vi "Bar Code Reader_v4.vi"() -> ()   [LabVIEW 2016]
uses:
  <vilib>/NXT/Block Support/NXT_OutputPort.ctl
  <vilib>/NXT/Block Support/NXT_InputPort.ctl
  <vilib>/NXT/Dual Mode Library/Sensors/EV3_Color_Color.vi
  <vilib>/NXT/NXTIO Xnodes/NXTIONodeSubVIs/NXTMoveMotors.vi
  <vilib>/NXT/NXTIO Xnodes/NXTIONodeSubVIs/NXTMotorRunDistance.vi
  <vilib>/NXT/Dual Mode Library/Waits/Wait_Num.vi
  <vilib>/NXT/Subs/LVHSConnector.ctl
  <vilib>/NXT/NXTIO Xnodes/AddressXNode/NXTIOAddress.xnode
  <vilib>/NXT/NXTIO Xnodes/NXTIOXNode/NXTIO.xnode
  <vilib>/NXT/LegoClasses/BrickReference/BrickReference.lvclass
panel:
  out "Error Message":string
  out "Total Marbles":dbl
  out "Small/HDPE 4":dbl
  out "Large/Steel 4":dbl
  out "Material 4":string
  out "Small/HDPE 3":dbl
  out "Large/Steel 3":dbl
  out "Material 3":string
  out "Small/HDPE 2":dbl
  out "Large/Steel 2":dbl
  out "Material 2":string
  out "Small/HDPE 1":dbl
  out "Large/Steel 1":dbl
  out "String 3":string
  out "String 2":string
  out "Material 1":string
  out "String":string
  out "Numeric":dbl
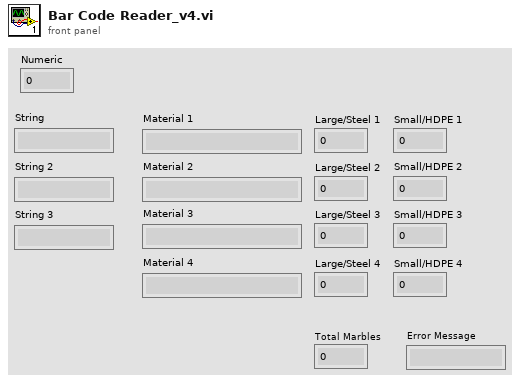
[diagram p1: front panel]
types:
  T1 = typedef "ColorSensorColors.ctl" = enum16{"No Color", "Black", "Blue", "Green", "Yellow", "Red", "White", "Brown"}
  T2 = typedef "NXT_OutputPort.ctl" = u8
  T3 = typedef "LVHSConnector.ctl" = refnum<class "BrickReference.lvclass">
  T4 = typedef "NXT_InputPort.ctl" = u32
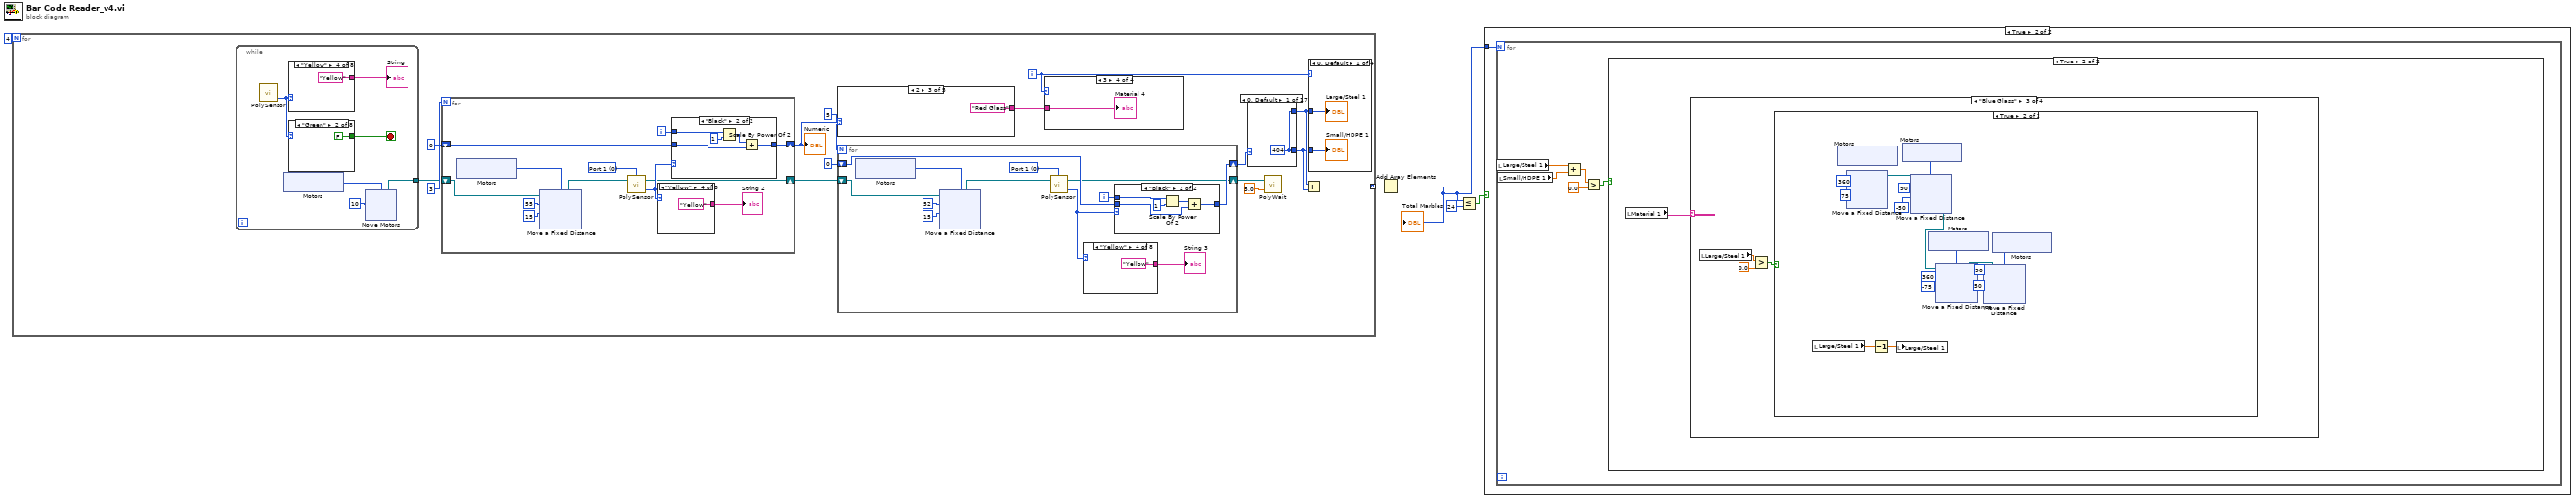
[diagram p0: block diagram]
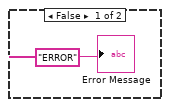
[diagram p2: hidden frame]
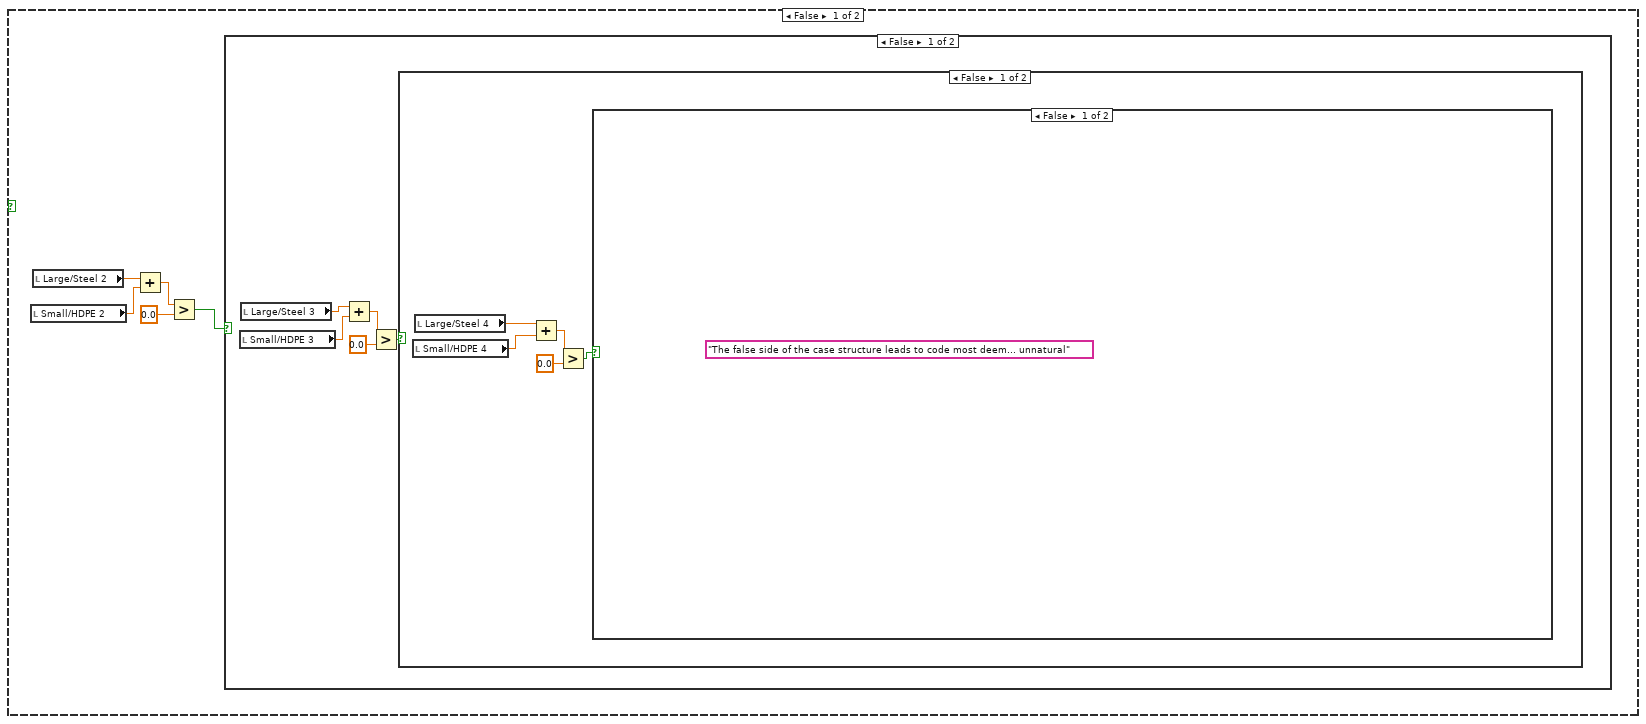
[diagram p3: hidden frame]
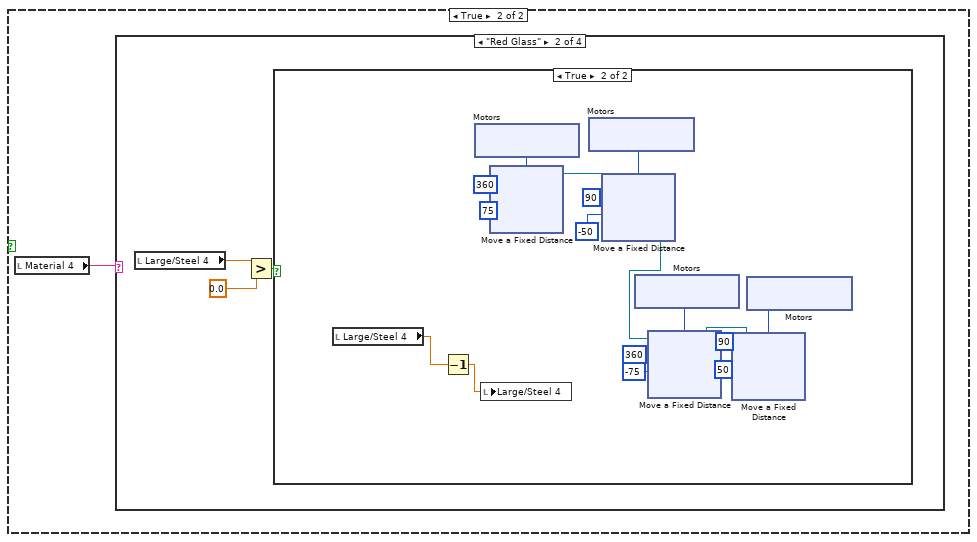
[diagram p4: hidden frame]
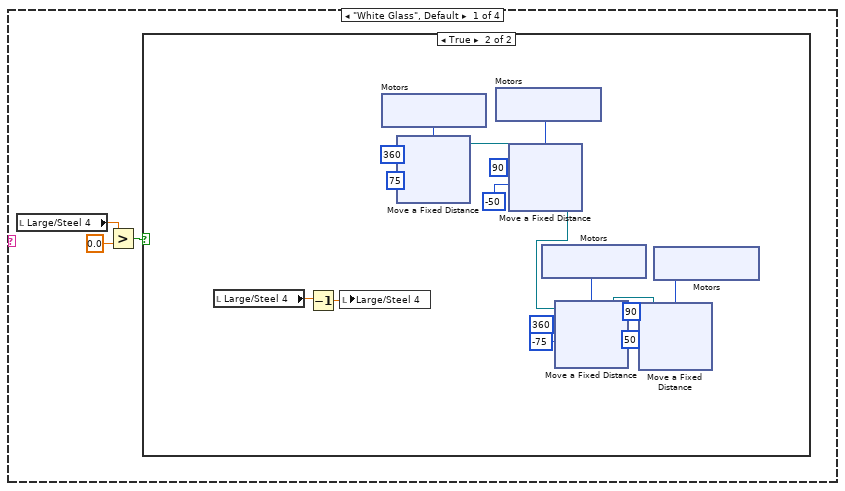
[diagram p5: hidden frame]
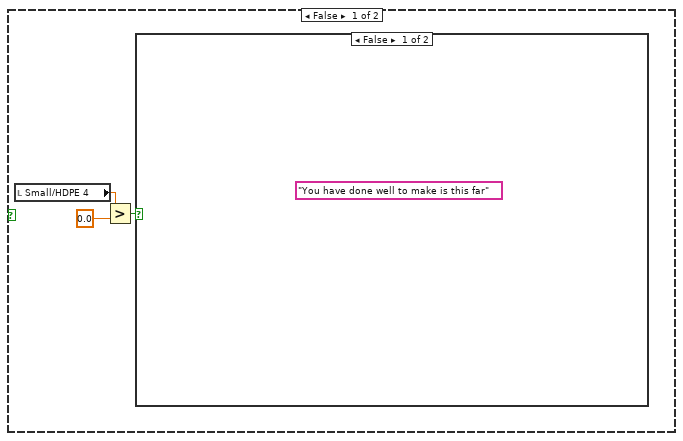
[diagram p6: hidden frame]
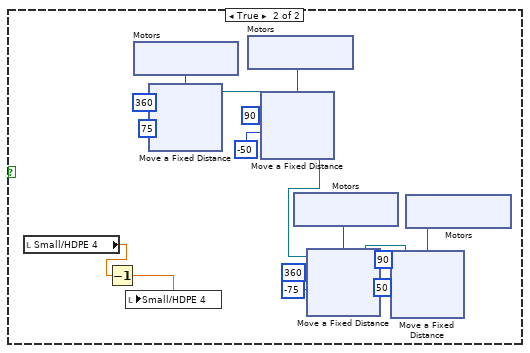
[diagram p7: hidden frame]
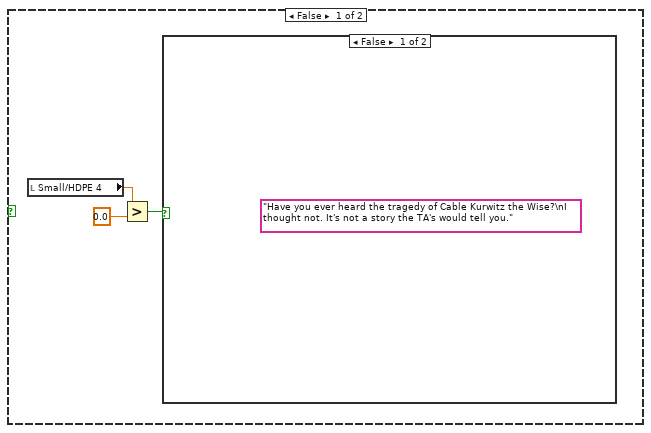
[diagram p8: hidden frame]
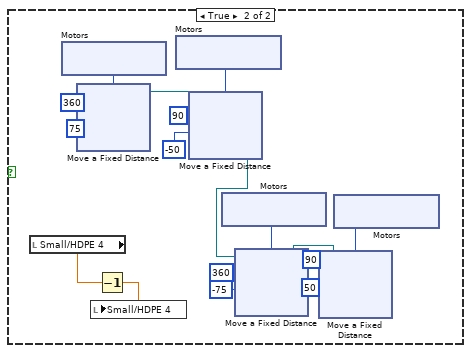
[diagram p9: hidden frame]
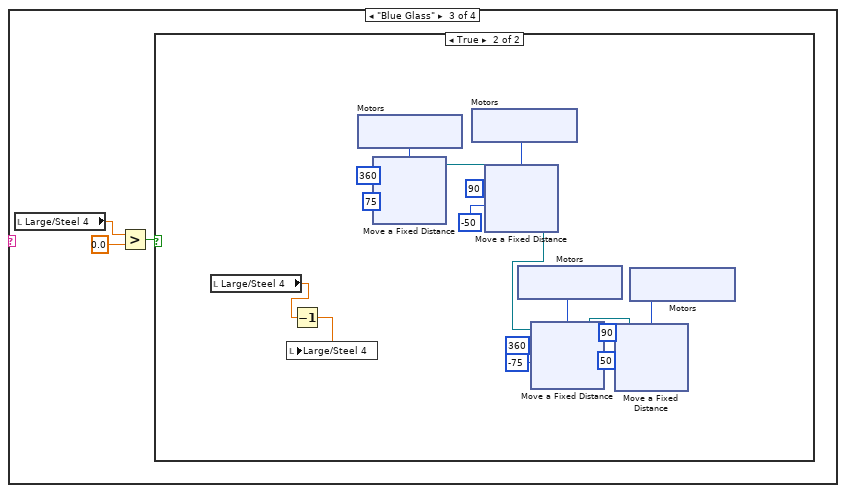
[diagram p10: hidden frame]
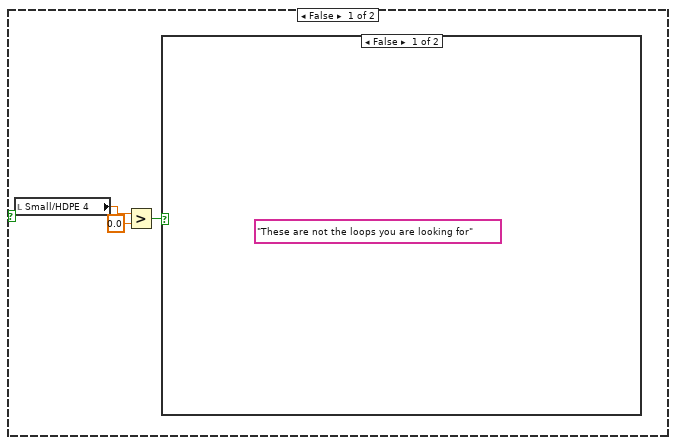
[diagram p11: hidden frame]
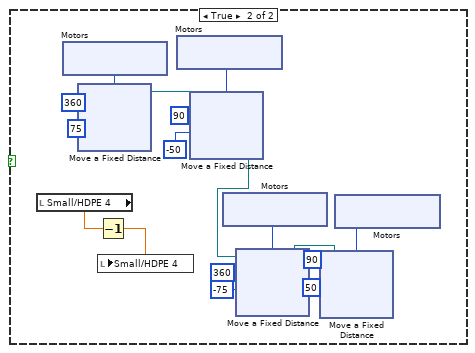
[diagram p12: hidden frame]
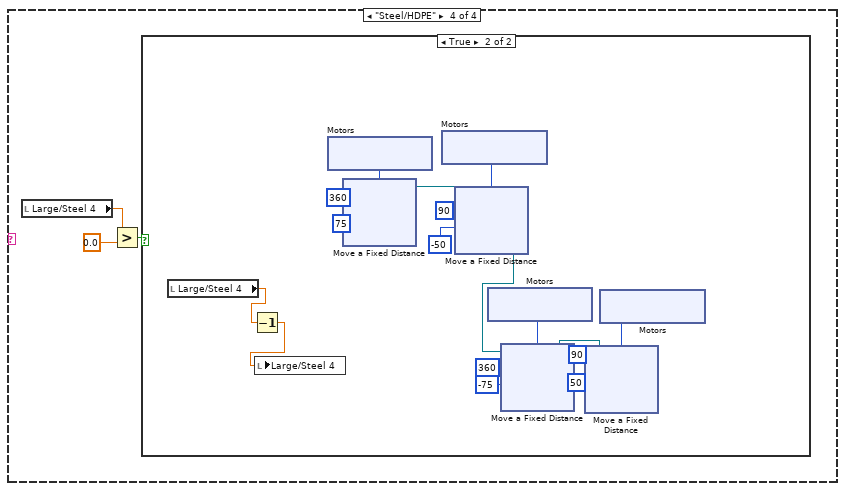
[diagram p13: hidden frame]
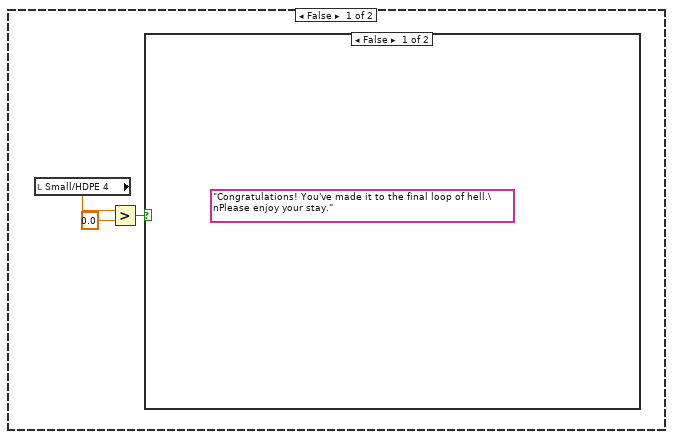
[diagram p14: hidden frame]
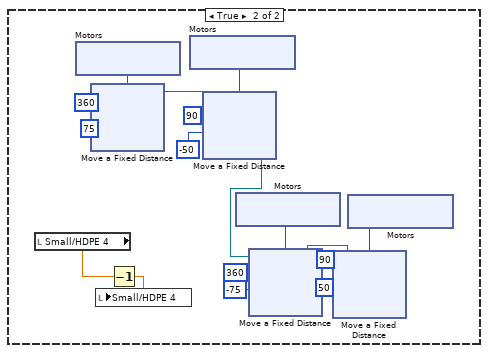
[diagram p15: hidden frame]
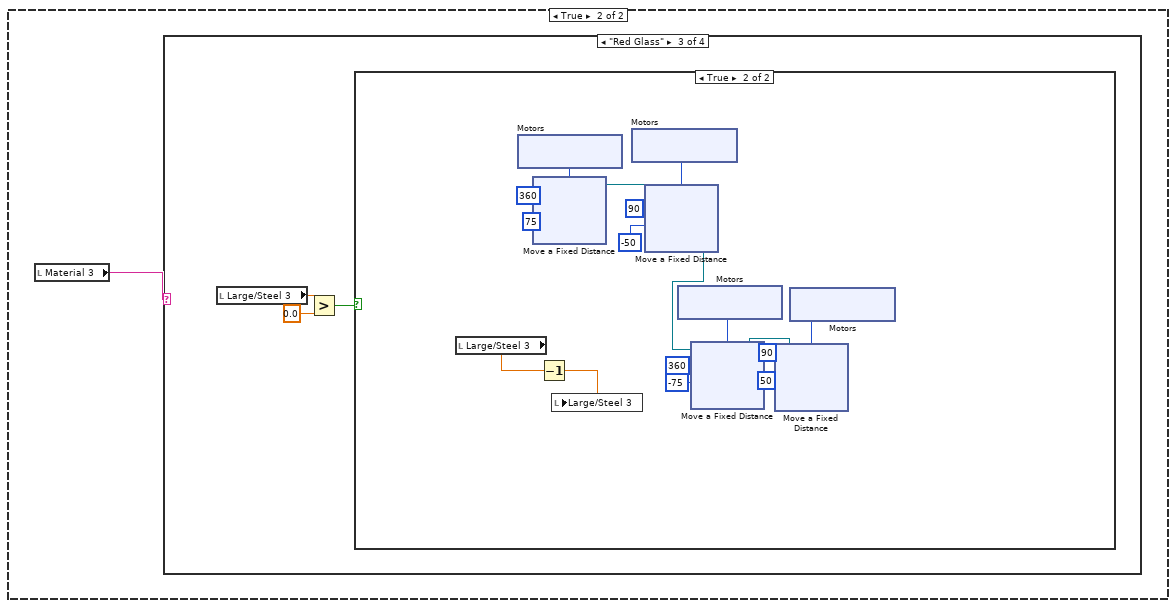
[diagram p16: hidden frame]
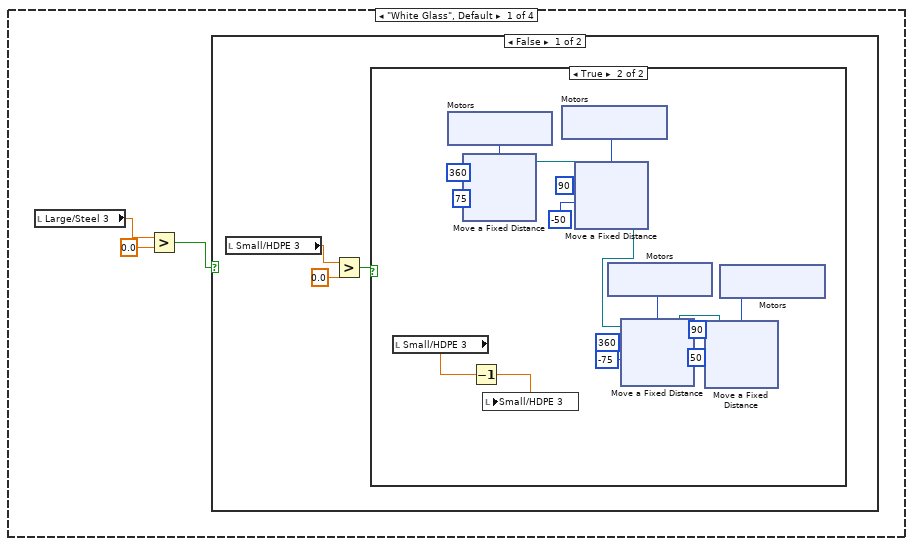
[diagram p17: hidden frame]
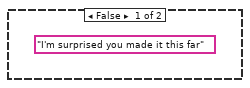
[diagram p18: hidden frame]
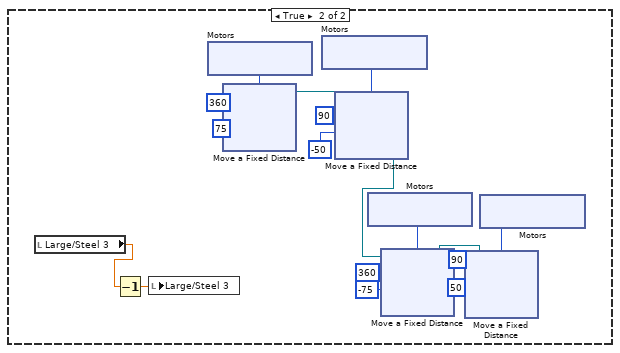
[diagram p19: hidden frame]
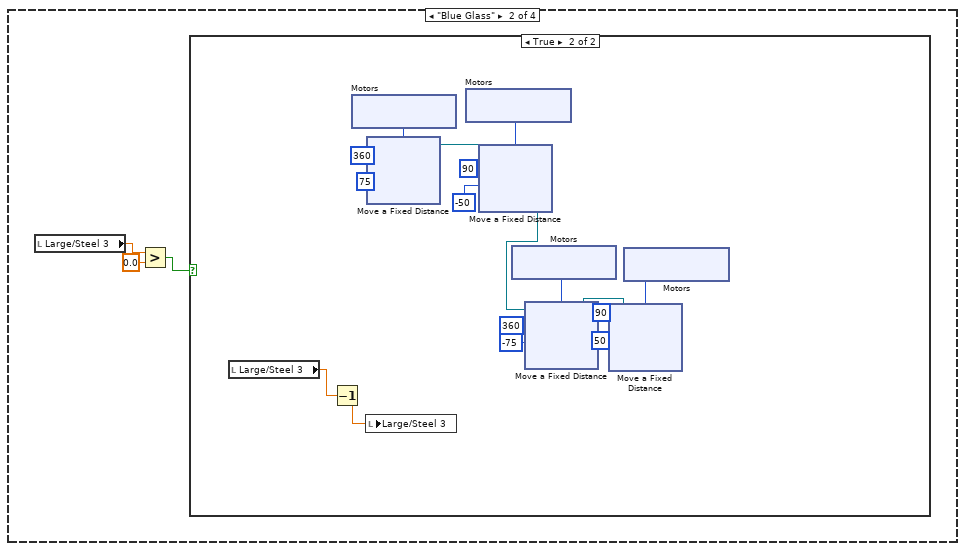
[diagram p20: hidden frame]
diagram:
  n1 = for {
    N: 4 -> [_]
    tunnel: [w6] -> w4 mode=indexing
    i -> [w11]
    n2 = while {
      tunnel: [w109] -> w18
      stop <- w113 stop-if-true
      n3 = call-poly <vilib>:"PolySensor.vi"() -> ("Detected Color"=w111:T1)  [unwired: 3 in, 1 out]
      n4 = xnode "Motors"() -> ("Motor"=w108:T2)
      n5 = case shown="\"Yellow\"" w111 {
        tunnel: ["No Color" "Blue" "Green" "Yellow" "Red" "White" "Brown" "Black"] -> w112
        frame "No Color", Default {
        }
        frame "Blue" {
        }
        frame "Green" {
        }
        frame "Yellow" {
        }
        frame "Red" {
        }
        frame "White" {
        }
        frame "Brown" {
        }
        frame "Black" {
        }
      }
      "String" <- w112
      n6 = case shown="\"Green\"" w111 {
        tunnel: [FALSE FALSE FALSE FALSE FALSE FALSE FALSE TRUE] -> w113
        frame "No Color", Default {
        }
        frame "Green" {
        }
        frame "Yellow" {
        }
        frame "Red" {
        }
        frame "White" {
        }
        frame "Brown" {
        }
        frame "Blue" {
        }
        frame "Black" {
        }
      }
      n7 = xnode "Move Motors"("Power/Speed 1"=i8 10, "Motors"=w108) -> ("NXT/EV3"=w109:T3)  [unwired: 1 in]
    }
    n8 = for {
      N: 3 -> [_]
      shift-right: [w149] -> w17
      shift-left: 0 -> [w148]
      shift-right: [w144] -> w13
      shift-left: w18 -> [w141]
      i -> [w145]
      w138 = T4 0 items=["Port 1", "Port 2", "Port 3", "Port 4"] ("Port (Port 1)")
      n9 = xnode "Motors"() -> ("Motor"=w139:T2)
      n10 = xnode "Move a Fixed Distance"("Speed 1"=i8 15, "Distance 1"=55, "Motors"=w139, "NXT/EV3"=w141) -> ("NXT/EV3"=w140:T3)
      n11 = call-poly <vilib>:"PolySensor.vi"("NXT/EV3"=w140, "Port (Port 1)"=w138) -> ("Detected Color"=w146:T1, "NXT/EV3"=w144:T3)  [unwired: 1 in]
      n12 = case shown="\"Yellow\"" w146 {
        tunnel: ["No Color" "Blue" "Green" "Yellow" "Red" "White" "Brown" "Black"] -> w147
        frame "No Color", Default {
        }
        frame "Blue" {
        }
        frame "Green" {
        }
        frame "Yellow" {
        }
        frame "Red" {
        }
        frame "White" {
        }
        frame "Brown" {
        }
        frame "Black" {
        }
      }
      "String 2" <- w147
      n13 = case shown="\"Black\"" w146 {
        tunnel: w145 -> [_ w173]
        tunnel: [w169 w171] -> w149
        tunnel: w148 -> [w169 w170]
        frame "White", Default {
        }
        frame "Black" {
          n14 = Scale By Power Of 2(n=w173, x=1) -> (x*2^n=w172:i32)
          n15 = Add(x=w172, y=w170) -> (x+y=w171:i32)
        }
      }
    }
    "Numeric" <- w17
    n16 = case shown="2" w17 {
      tunnel: ["Something has gone wrong" "White Glass" "Red Glass" "Blue Glass" "Steel/HDPE"] -> w16
      frame 0, Default {
      }
      frame 1 {
      }
      frame 2 {
      }
      frame 3 {
      }
      frame 4 {
      }
    }
    n17 = for {
      N: 5 -> [_]
      shift-right: [w77] -> w12
      shift-left: 0 -> [w76]
      shift-right: [w72] -> w10
      shift-left: w13 -> [w69]
      i -> [w73]
      w66 = T4 0 items=["Port 1", "Port 2", "Port 3", "Port 4"] ("Port (Port 1)")
      n18 = xnode "Motors"() -> ("Motor"=w67:T2)
      n19 = xnode "Move a Fixed Distance"("Speed 1"=i8 15, "Distance 1"=52, "Motors"=w67, "NXT/EV3"=w69) -> ("NXT/EV3"=w68:T3)
      n20 = call-poly <vilib>:"PolySensor.vi"("NXT/EV3"=w68, "Port (Port 1)"=w66) -> ("Detected Color"=w74:T1, "NXT/EV3"=w72:T3)  [unwired: 1 in]
      n21 = case shown="\"Yellow\"" w74 {
        tunnel: ["No Color" "Blue" "Green" "Yellow" "Red" "White" "Brown" "Black"] -> w75
        frame "No Color", Default {
        }
        frame "Blue" {
        }
        frame "Green" {
        }
        frame "Yellow" {
        }
        frame "Red" {
        }
        frame "White" {
        }
        frame "Brown" {
        }
        frame "Black" {
        }
      }
      "String 3" <- w75
      n22 = case shown="\"Black\"" w74 {
        tunnel: w73 -> [_ w101]
        tunnel: [w97 w99] -> w77
        tunnel: w76 -> [w97 w98]
        frame "White", Default {
        }
        frame "Black" {
          n23 = Scale By Power Of 2(n=w101, x=1) -> (x*2^n=w100:i32)
          n24 = Add(x=w100, y=w98) -> (x+y=w99:i32)
        }
      }
    }
    n25 = case shown="3" w11 {
      tunnel: w16 -> [w29 w30 w31 w32]
      frame 0, Default {
        "Material 1" <- w29
      }
      frame 1 {
        "Material 2" <- w30
      }
      frame 2 {
        "Material 3" <- w31
      }
      frame 3 {
        "Material 4" <- w32
      }
    }
    n26 = case shown="0, Default" w12 {
      tunnel: [w33 0 1 2 3 0 1 2 3 0 1 2 3 0 1 2 3] -> w8
      tunnel: [w33 0 0 0 0 1 1 1 1 2 2 2 2 3 3 3 3] -> w7
      frame 0, Default {
        w33 = 404
      }
      frame 1 {
      }
      frame 2 {
      }
      frame 3 {
      }
      frame 4 {
      }
      frame 5 {
      }
      frame 6 {
      }
      frame 7 {
      }
      frame 8 {
      }
      frame 9 {
      }
      frame 10 {
      }
      frame 11 {
      }
      frame 12 {
      }
      frame 13 {
      }
      frame 14 {
      }
      frame 15 {
      }
      frame 16 {
      }
    }
    n27 = call-poly <vilib>:"PolyWait.vi"("Time (1 sec)"=sgl 5.0, "NXT/EV3"=w10) -> ()  [unwired: 2 in, 1 out]
    n28 = Add(x=w8, y=w7) -> (x+y=w6:i32)
    n29 = case shown="0, Default" w11 {
      tunnel: w8 -> [w22 w23 w25 w27]
      tunnel: w7 -> [w21 w24 w26 w28]
      frame 0, Default {
        "Small/HDPE 1" <- w21
        "Large/Steel 1" <- w22
      }
      frame 1 {
        "Large/Steel 2" <- w23
        "Small/HDPE 2" <- w24
      }
      frame 2 {
        "Large/Steel 3" <- w25
        "Small/HDPE 3" <- w26
      }
      frame 3 {
        "Large/Steel 4" <- w27
        "Small/HDPE 4" <- w28
      }
    }
  }
  n30 = Add Array Elements(numeric array=w4) -> (sum=w3:i32)
  "Total Marbles" <- w3
  n31 = Less Or Equal?(x=w3, y=24) -> (x <= y?=w1:bool)
  n32 = case shown="True" w1 {
    tunnel: w3 -> [_ w176]
    frame False {
      "Error Message" <- "ERROR"
    }
    frame True {
      n33 = for {
        N: w176 -> [_]
        n34 = local read "Large/Steel 1"() -> (w181:dbl)
        n35 = local read "Small/HDPE 1"() -> (w180:dbl)
        n36 = Add(x=w181, y=w180) -> (x+y=w179:dbl)
        n37 = Greater?(x=w179, y=0.0) -> (0:w177:bool)
        n38 = case shown="True" w177 {
          frame False {
            n39 = local read "Small/HDPE 2"() -> (w184:dbl)
            n40 = local read "Large/Steel 2"() -> (w183:dbl)
            n41 = Add(x=w183, y=w184) -> (x+y=w186:dbl)
            n42 = Greater?(x=w186, y=0.0) -> (0:w182:bool)
            n43 = case shown="False" w182 {
              frame False {
                n44 = local read "Small/HDPE 3"() -> (w188:dbl)
                n45 = local read "Large/Steel 3"() -> (w189:dbl)
                n46 = Add(x=w189, y=w188) -> (x+y=w191:dbl)
                n47 = Greater?(x=w191, y=0.0) -> (0:w187:bool)
                n48 = case shown="False" w187 {
                  frame False {
                    n49 = local read "Small/HDPE 4"() -> (w193:dbl)
                    n50 = local read "Large/Steel 4"() -> (w194:dbl)
                    n51 = Add(x=w194, y=w193) -> (x+y=w196:dbl)
                    n52 = Greater?(x=w196, y=0.0) -> (0:w192:bool)
                    n53 = case shown="False" w192 {
                      frame False {
                        (unwired) "The false side of the case structure leads to code most deem... unnatural"
                      }
                      frame True {
                        n54 = local read "Material 4"() -> (w197:string)
                        n55 = case shown="\"Red Glass\"" w197 {
                          frame "White Glass", Default {
                            n56 = local read "Large/Steel 4"() -> (w199:dbl)
                            n57 = Greater?(x=w199, y=0.0) -> (0:w200:bool)
                            n58 = case shown="True" w200 {
                              frame False {
                                n59 = local read "Small/HDPE 4"() -> (w202:dbl)
                                n60 = Greater?(x=w202, y=0.0) -> (0:w203:bool)
                                n61 = case shown="False" w203 {
                                frame False {
                                (unwired) "You have done well to make is this far"
                                }
                                frame True {
                                n62 = local read "Small/HDPE 4"() -> (w220:dbl)
                                n63 = Decrement(x=w220) -> (x-1=w219:dbl)
                                n64 = local write "Small/HDPE 4"(w219) -> ()
                                n65 = xnode "Motors"() -> ("Motor"=w204:T2)
                                n66 = xnode "Move a Fixed Distance"("Speed 1"=i8 75, "Distance 1"=360, "Motors"=w204) -> ("NXT/EV3"=w207:T3)  [unwired: 1 in]
                                n67 = xnode "Motors"() -> ("Motor"=w208:T2)
                                n68 = xnode "Move a Fixed Distance"("Speed 1"=i8 -50, "Distance 1"=90, "Motors"=w208, "NXT/EV3"=w207) -> ("NXT/EV3"=w218:T3)
                                n69 = xnode "Motors"() -> ("Motor"=w214:T2)
                                n70 = xnode "Move a Fixed Distance"("Speed 1"=i8 -75, "Distance 1"=360, "Motors"=w214, "NXT/EV3"=w218) -> ("NXT/EV3"=w217:T3)
                                n71 = xnode "Motors"() -> ("Motor"=w211:T2)
                                n72 = xnode "Move a Fixed Distance"("Speed 1"=i8 50, "Distance 1"=90, "Motors"=w211, "NXT/EV3"=w217) -> ()  [unwired: 1 out]
                                }
                                }
                              }
                              frame True {
                                n73 = local read "Large/Steel 4"() -> (w281:dbl)
                                n74 = Decrement(x=w281) -> (x-1=w280:dbl)
                                n75 = local write "Large/Steel 4"(w280) -> ()
                                n76 = xnode "Motors"() -> ("Motor"=w265:T2)
                                n77 = xnode "Move a Fixed Distance"("Speed 1"=i8 75, "Distance 1"=360, "Motors"=w265) -> ("NXT/EV3"=w268:T3)  [unwired: 1 in]
                                n78 = xnode "Motors"() -> ("Motor"=w269:T2)
                                n79 = xnode "Move a Fixed Distance"("Speed 1"=i8 -50, "Distance 1"=90, "Motors"=w269, "NXT/EV3"=w268) -> ("NXT/EV3"=w279:T3)
                                n80 = xnode "Motors"() -> ("Motor"=w275:T2)
                                n81 = xnode "Move a Fixed Distance"("Speed 1"=i8 -75, "Distance 1"=360, "Motors"=w275, "NXT/EV3"=w279) -> ("NXT/EV3"=w278:T3)
                                n82 = xnode "Motors"() -> ("Motor"=w272:T2)
                                n83 = xnode "Move a Fixed Distance"("Speed 1"=i8 50, "Distance 1"=90, "Motors"=w272, "NXT/EV3"=w278) -> ()  [unwired: 1 out]
                              }
                            }
                          }
                          frame "Red Glass" {
                            n84 = local read "Large/Steel 4"() -> (w327:dbl)
                            n85 = Greater?(x=w327, y=0.0) -> (0:w328:bool)
                            n86 = case shown="True" w328 {
                              frame False {
                                n87 = local read "Small/HDPE 4"() -> (w329:dbl)
                                n88 = Greater?(x=w329, y=0.0) -> (0:w331:bool)
                                n89 = case shown="False" w331 {
                                frame False {
                                (unwired) "Have you ever heard the tragedy of Cable Kurwitz the Wise?\nI thought not. It's not a story the TA's would tell you."
                                }
                                frame True {
                                n90 = local read "Small/HDPE 4"() -> (w348:dbl)
                                n91 = xnode "Motors"() -> ("Motor"=w332:T2)
                                n92 = xnode "Move a Fixed Distance"("Speed 1"=i8 75, "Distance 1"=360, "Motors"=w332) -> ("NXT/EV3"=w335:T3)  [unwired: 1 in]
                                n93 = Decrement(x=w348) -> (x-1=w347:dbl)
                                n94 = local write "Small/HDPE 4"(w347) -> ()
                                n95 = xnode "Motors"() -> ("Motor"=w336:T2)
                                n96 = xnode "Move a Fixed Distance"("Speed 1"=i8 -50, "Distance 1"=90, "Motors"=w336, "NXT/EV3"=w335) -> ("NXT/EV3"=w346:T3)
                                n97 = xnode "Motors"() -> ("Motor"=w342:T2)
                                n98 = xnode "Move a Fixed Distance"("Speed 1"=i8 -75, "Distance 1"=360, "Motors"=w342, "NXT/EV3"=w346) -> ("NXT/EV3"=w345:T3)
                                n99 = xnode "Motors"() -> ("Motor"=w339:T2)
                                n100 = xnode "Move a Fixed Distance"("Speed 1"=i8 50, "Distance 1"=90, "Motors"=w339, "NXT/EV3"=w345) -> ()  [unwired: 1 out]
                                }
                                }
                              }
                              frame True {
                                n101 = local read "Large/Steel 4"() -> (w409:dbl)
                                n102 = Decrement(x=w409) -> (x-1=w408:dbl)
                                n103 = xnode "Motors"() -> ("Motor"=w393:T2)
                                n104 = local write "Large/Steel 4"(w408) -> ()
                                n105 = xnode "Move a Fixed Distance"("Speed 1"=i8 75, "Distance 1"=360, "Motors"=w393) -> ("NXT/EV3"=w396:T3)  [unwired: 1 in]
                                n106 = xnode "Motors"() -> ("Motor"=w397:T2)
                                n107 = xnode "Move a Fixed Distance"("Speed 1"=i8 -50, "Distance 1"=90, "Motors"=w397, "NXT/EV3"=w396) -> ("NXT/EV3"=w407:T3)
                                n108 = xnode "Motors"() -> ("Motor"=w403:T2)
                                n109 = xnode "Move a Fixed Distance"("Speed 1"=i8 -75, "Distance 1"=360, "Motors"=w403, "NXT/EV3"=w407) -> ("NXT/EV3"=w406:T3)
                                n110 = xnode "Motors"() -> ("Motor"=w400:T2)
                                n111 = xnode "Move a Fixed Distance"("Speed 1"=i8 50, "Distance 1"=90, "Motors"=w400, "NXT/EV3"=w406) -> ()  [unwired: 1 out]
                              }
                            }
                          }
                          frame "Blue Glass" {
                            n112 = local read "Large/Steel 4"() -> (w456:dbl)
                            n113 = Greater?(x=w456, y=0.0) -> (0:w455:bool)
                            n114 = case shown="True" w455 {
                              frame False {
                                n115 = local read "Small/HDPE 4"() -> (w458:dbl)
                                n116 = Greater?(x=w458, y=0.0) -> (0:w459:bool)
                                n117 = case shown="False" w459 {
                                frame False {
                                (unwired) "These are not the loops you are looking for"
                                }
                                frame True {
                                n118 = local read "Small/HDPE 4"() -> (w476:dbl)
                                n119 = xnode "Motors"() -> ("Motor"=w460:T2)
                                n120 = xnode "Move a Fixed Distance"("Speed 1"=i8 75, "Distance 1"=360, "Motors"=w460) -> ("NXT/EV3"=w463:T3)  [unwired: 1 in]
                                n121 = Decrement(x=w476) -> (x-1=w475:dbl)
                                n122 = local write "Small/HDPE 4"(w475) -> ()
                                n123 = xnode "Motors"() -> ("Motor"=w464:T2)
                                n124 = xnode "Move a Fixed Distance"("Speed 1"=i8 -50, "Distance 1"=90, "Motors"=w464, "NXT/EV3"=w463) -> ("NXT/EV3"=w474:T3)
                                n125 = xnode "Motors"() -> ("Motor"=w470:T2)
                                n126 = xnode "Move a Fixed Distance"("Speed 1"=i8 -75, "Distance 1"=360, "Motors"=w470, "NXT/EV3"=w474) -> ("NXT/EV3"=w473:T3)
                                n127 = xnode "Motors"() -> ("Motor"=w467:T2)
                                n128 = xnode "Move a Fixed Distance"("Speed 1"=i8 50, "Distance 1"=90, "Motors"=w467, "NXT/EV3"=w473) -> ()  [unwired: 1 out]
                                }
                                }
                              }
                              frame True {
                                n129 = local read "Large/Steel 4"() -> (w537:dbl)
                                n130 = Decrement(x=w537) -> (x-1=w536:dbl)
                                n131 = local write "Large/Steel 4"(w536) -> ()
                                n132 = xnode "Motors"() -> ("Motor"=w521:T2)
                                n133 = xnode "Move a Fixed Distance"("Speed 1"=i8 75, "Distance 1"=360, "Motors"=w521) -> ("NXT/EV3"=w524:T3)  [unwired: 1 in]
                                n134 = xnode "Motors"() -> ("Motor"=w525:T2)
                                n135 = xnode "Move a Fixed Distance"("Speed 1"=i8 -50, "Distance 1"=90, "Motors"=w525, "NXT/EV3"=w524) -> ("NXT/EV3"=w535:T3)
                                n136 = xnode "Motors"() -> ("Motor"=w531:T2)
                                n137 = xnode "Move a Fixed Distance"("Speed 1"=i8 -75, "Distance 1"=360, "Motors"=w531, "NXT/EV3"=w535) -> ("NXT/EV3"=w534:T3)
                                n138 = xnode "Motors"() -> ("Motor"=w528:T2)
                                n139 = xnode "Move a Fixed Distance"("Speed 1"=i8 50, "Distance 1"=90, "Motors"=w528, "NXT/EV3"=w534) -> ()  [unwired: 1 out]
                              }
                            }
                          }
                          frame "Steel/HDPE" {
                            n140 = local read "Large/Steel 4"() -> (w583:dbl)
                            n141 = Greater?(x=w583, y=0.0) -> (0:w584:bool)
                            n142 = case shown="True" w584 {
                              frame False {
                                n143 = local read "Small/HDPE 4"() -> (w586:dbl)
                                n144 = Greater?(x=w586, y=0.0) -> (0:w587:bool)
                                n145 = case shown="False" w587 {
                                frame False {
                                (unwired) "Congratulations! You've made it to the final loop of hell.\nPlease enjoy your stay."
                                }
                                frame True {
                                n146 = local read "Small/HDPE 4"() -> (w604:dbl)
                                n147 = xnode "Motors"() -> ("Motor"=w588:T2)
                                n148 = xnode "Move a Fixed Distance"("Speed 1"=i8 75, "Distance 1"=360, "Motors"=w588) -> ("NXT/EV3"=w591:T3)  [unwired: 1 in]
                                n149 = Decrement(x=w604) -> (x-1=w603:dbl)
                                n150 = local write "Small/HDPE 4"(w603) -> ()
                                n151 = xnode "Motors"() -> ("Motor"=w592:T2)
                                n152 = xnode "Move a Fixed Distance"("Speed 1"=i8 -50, "Distance 1"=90, "Motors"=w592, "NXT/EV3"=w591) -> ("NXT/EV3"=w602:T3)
                                n153 = xnode "Motors"() -> ("Motor"=w598:T2)
                                n154 = xnode "Move a Fixed Distance"("Speed 1"=i8 -75, "Distance 1"=360, "Motors"=w598, "NXT/EV3"=w602) -> ("NXT/EV3"=w601:T3)
                                n155 = xnode "Motors"() -> ("Motor"=w595:T2)
                                n156 = xnode "Move a Fixed Distance"("Speed 1"=i8 50, "Distance 1"=90, "Motors"=w595, "NXT/EV3"=w601) -> ()  [unwired: 1 out]
                                }
                                }
                              }
                              frame True {
                                n157 = local read "Large/Steel 4"() -> (w665:dbl)
                                n158 = Decrement(x=w665) -> (x-1=w664:dbl)
                                n159 = local write "Large/Steel 4"(w664) -> ()
                                n160 = xnode "Motors"() -> ("Motor"=w649:T2)
                                n161 = xnode "Move a Fixed Distance"("Speed 1"=i8 75, "Distance 1"=360, "Motors"=w649) -> ("NXT/EV3"=w652:T3)  [unwired: 1 in]
                                n162 = xnode "Motors"() -> ("Motor"=w653:T2)
                                n163 = xnode "Move a Fixed Distance"("Speed 1"=i8 -50, "Distance 1"=90, "Motors"=w653, "NXT/EV3"=w652) -> ("NXT/EV3"=w663:T3)
                                n164 = xnode "Motors"() -> ("Motor"=w659:T2)
                                n165 = xnode "Move a Fixed Distance"("Speed 1"=i8 -75, "Distance 1"=360, "Motors"=w659, "NXT/EV3"=w663) -> ("NXT/EV3"=w662:T3)
                                n166 = xnode "Motors"() -> ("Motor"=w656:T2)
                                n167 = xnode "Move a Fixed Distance"("Speed 1"=i8 50, "Distance 1"=90, "Motors"=w656, "NXT/EV3"=w662) -> ()  [unwired: 1 out]
                              }
                            }
                          }
                        }
                      }
                    }
                  }
                  frame True {
                    n168 = local read "Material 3"() -> (w710:string)
                    n169 = case shown="\"Red Glass\"" w710 {
                      frame "White Glass", Default {
                        n170 = local read "Large/Steel 3"() -> (w713:dbl)
                        n171 = Greater?(x=w713, y=0.0) -> (0:w711:bool)
                        n172 = case shown="False" w711 {
                          frame False {
                            n173 = local read "Small/HDPE 3"() -> (w715:dbl)
                            n174 = Greater?(x=w715, y=0.0) -> (0:w716:bool)
                            n175 = case shown="True" w716 {
                              frame False {
                                (unwired) "I'm surprised you made it this far"
                              }
                              frame True {
                                n176 = local read "Small/HDPE 3"() -> (w733:dbl)
                                n177 = xnode "Motors"() -> ("Motor"=w717:T2)
                                n178 = xnode "Move a Fixed Distance"("Speed 1"=i8 75, "Distance 1"=360, "Motors"=w717) -> ("NXT/EV3"=w720:T3)  [unwired: 1 in]
                                n179 = Decrement(x=w733) -> (x-1=w732:dbl)
                                n180 = local write "Small/HDPE 3"(w732) -> ()
                                n181 = xnode "Motors"() -> ("Motor"=w721:T2)
                                n182 = xnode "Move a Fixed Distance"("Speed 1"=i8 -50, "Distance 1"=90, "Motors"=w721, "NXT/EV3"=w720) -> ("NXT/EV3"=w731:T3)
                                n183 = xnode "Motors"() -> ("Motor"=w727:T2)
                                n184 = xnode "Move a Fixed Distance"("Speed 1"=i8 -75, "Distance 1"=360, "Motors"=w727, "NXT/EV3"=w731) -> ("NXT/EV3"=w730:T3)
                                n185 = xnode "Motors"() -> ("Motor"=w724:T2)
                                n186 = xnode "Move a Fixed Distance"("Speed 1"=i8 50, "Distance 1"=90, "Motors"=w724, "NXT/EV3"=w730) -> ()  [unwired: 1 out]
                              }
                            }
                          }
                          frame True {
                            n187 = local read "Large/Steel 3"() -> (w794:dbl)
                            n188 = Decrement(x=w794) -> (x-1=w793:dbl)
                            n189 = local write "Large/Steel 3"(w793) -> ()
                            n190 = xnode "Motors"() -> ("Motor"=w778:T2)
                            n191 = xnode "Move a Fixed Distance"("Speed 1"=i8 75, "Distance 1"=360, "Motors"=w778) -> ("NXT/EV3"=w781:T3)  [unwired: 1 in]
                            n192 = xnode "Motors"() -> ("Motor"=w782:T2)
                            n193 = xnode "Move a Fixed Distance"("Speed 1"=i8 -50, "Distance 1"=90, "Motors"=w782, "NXT/EV3"=w781) -> ("NXT/EV3"=w792:T3)
                            n194 = xnode "Motors"() -> ("Motor"=w788:T2)
                            n195 = xnode "Move a Fixed Distance"("Speed 1"=i8 -75, "Distance 1"=360, "Motors"=w788, "NXT/EV3"=w792) -> ("NXT/EV3"=w791:T3)
                            n196 = xnode "Motors"() -> ("Motor"=w785:T2)
                            n197 = xnode "Move a Fixed Distance"("Speed 1"=i8 50, "Distance 1"=90, "Motors"=w785, "NXT/EV3"=w791) -> ()  [unwired: 1 out]
                          }
                        }
                      }
                      frame "Blue Glass" {
                        n198 = local read "Large/Steel 3"() -> (w841:dbl)
                        n199 = Greater?(x=w841, y=0.0) -> (0:w839:bool)
                        n200 = case shown="True" w839 {
                          frame False {
                            n201 = local read "Small/HDPE 3"() -> (w844:dbl)
                            n202 = Greater?(x=w844, y=0.0) -> (0:w842:bool)
                            n203 = case shown="False" w842 {
                              frame False {
                                (unwired) "Welcome to the dark side of the case structure"
                              }
                              frame True {
                                n204 = local read "Small/HDPE 3"() -> (w861:dbl)
                                n205 = xnode "Motors"() -> ("Motor"=w845:T2)
                                n206 = Decrement(x=w861) -> (x-1=w860:dbl)
                                n207 = xnode "Move a Fixed Distance"("Speed 1"=i8 75, "Distance 1"=360, "Motors"=w845) -> ("NXT/EV3"=w848:T3)  [unwired: 1 in]
                                n208 = local write "Small/HDPE 3"(w860) -> ()
                                n209 = xnode "Motors"() -> ("Motor"=w849:T2)
                                n210 = xnode "Move a Fixed Distance"("Speed 1"=i8 -50, "Distance 1"=90, "Motors"=w849, "NXT/EV3"=w848) -> ("NXT/EV3"=w859:T3)
                                n211 = xnode "Motors"() -> ("Motor"=w855:T2)
                                n212 = xnode "Move a Fixed Distance"("Speed 1"=i8 -75, "Distance 1"=360, "Motors"=w855, "NXT/EV3"=w859) -> ("NXT/EV3"=w858:T3)
                                n213 = xnode "Motors"() -> ("Motor"=w852:T2)
                                n214 = xnode "Move a Fixed Distance"("Speed 1"=i8 50, "Distance 1"=90, "Motors"=w852, "NXT/EV3"=w858) -> ()  [unwired: 1 out]
                              }
                            }
                          }
                          frame True {
                            n215 = local read "Large/Steel 3"() -> (w922:dbl)
                            n216 = Decrement(x=w922) -> (x-1=w921:dbl)
                            n217 = xnode "Motors"() -> ("Motor"=w906:T2)
                            n218 = local write "Large/Steel 3"(w921) -> ()
                            n219 = xnode "Move a Fixed Distance"("Speed 1"=i8 75, "Distance 1"=360, "Motors"=w906) -> ("NXT/EV3"=w909:T3)  [unwired: 1 in]
                            n220 = xnode "Motors"() -> ("Motor"=w910:T2)
                            n221 = xnode "Move a Fixed Distance"("Speed 1"=i8 -50, "Distance 1"=90, "Motors"=w910, "NXT/EV3"=w909) -> ("NXT/EV3"=w920:T3)
                            n222 = xnode "Motors"() -> ("Motor"=w916:T2)
                            n223 = xnode "Move a Fixed Distance"("Speed 1"=i8 -75, "Distance 1"=360, "Motors"=w916, "NXT/EV3"=w920) -> ("NXT/EV3"=w919:T3)
                            n224 = xnode "Motors"() -> ("Motor"=w913:T2)
                            n225 = xnode "Move a Fixed Distance"("Speed 1"=i8 50, "Distance 1"=90, "Motors"=w913, "NXT/EV3"=w919) -> ()  [unwired: 1 out]
                          }
                        }
                      }
                      frame "Red Glass" {
                        n226 = local read "Large/Steel 3"() -> (w968:dbl)
                        n227 = Greater?(x=w968, y=0.0) -> (0:w969:bool)
                        n228 = case shown="True" w969 {
                          frame False {
                            n229 = local read "Small/HDPE 3"() -> (w971:dbl)
                            n230 = Greater?(x=w971, y=0.0) -> (0:w972:bool)
                            n231 = case shown="False" w972 {
                              frame False {
                                (unwired) "Two to the one to the one to the three"
                              }
                              frame True {
                                n232 = local read "Small/HDPE 3"() -> (w989:dbl)
                                n233 = Decrement(x=w989) -> (x-1=w988:dbl)
                                n234 = local write "Small/HDPE 3"(w988) -> ()
                                n235 = xnode "Motors"() -> ("Motor"=w973:T2)
                                n236 = xnode "Move a Fixed Distance"("Speed 1"=i8 75, "Distance 1"=360, "Motors"=w973) -> ("NXT/EV3"=w976:T3)  [unwired: 1 in]
                                n237 = xnode "Motors"() -> ("Motor"=w977:T2)
                                n238 = xnode "Move a Fixed Distance"("Speed 1"=i8 -50, "Distance 1"=90, "Motors"=w977, "NXT/EV3"=w976) -> ("NXT/EV3"=w987:T3)
                                n239 = xnode "Motors"() -> ("Motor"=w983:T2)
                                n240 = xnode "Move a Fixed Distance"("Speed 1"=i8 -75, "Distance 1"=360, "Motors"=w983, "NXT/EV3"=w987) -> ("NXT/EV3"=w986:T3)
                                n241 = xnode "Motors"() -> ("Motor"=w980:T2)
                                n242 = xnode "Move a Fixed Distance"("Speed 1"=i8 50, "Distance 1"=90, "Motors"=w980, "NXT/EV3"=w986) -> ()  [unwired: 1 out]
                              }
                            }
                          }
                          frame True {
                            n243 = local read "Large/Steel 3"() -> (w1050:dbl)
                            n244 = xnode "Motors"() -> ("Motor"=w1034:T2)
                            n245 = xnode "Move a Fixed Distance"("Speed 1"=i8 75, "Distance 1"=360, "Motors"=w1034) -> ("NXT/EV3"=w1037:T3)  [unwired: 1 in]
                            n246 = Decrement(x=w1050) -> (x-1=w1049:dbl)
                            n247 = local write "Large/Steel 3"(w1049) -> ()
                            n248 = xnode "Motors"() -> ("Motor"=w1038:T2)
                            n249 = xnode "Move a Fixed Distance"("Speed 1"=i8 -50, "Distance 1"=90, "Motors"=w1038, "NXT/EV3"=w1037) -> ("NXT/EV3"=w1048:T3)
                            n250 = xnode "Motors"() -> ("Motor"=w1044:T2)
                            n251 = xnode "Move a Fixed Distance"("Speed 1"=i8 -75, "Distance 1"=360, "Motors"=w1044, "NXT/EV3"=w1048) -> ("NXT/EV3"=w1047:T3)
                            n252 = xnode "Motors"() -> ("Motor"=w1041:T2)
                            n253 = xnode "Move a Fixed Distance"("Speed 1"=i8 50, "Distance 1"=90, "Motors"=w1041, "NXT/EV3"=w1047) -> ()  [unwired: 1 out]
                          }
                        }
                      }
                      frame "Steel/HDPE" {
                        n254 = local read "Large/Steel 3"() -> (w1096:dbl)
                        n255 = Greater?(x=w1096, y=0.0) -> (0:w1097:bool)
                        n256 = case shown="True" w1097 {
                          frame False {
                            n257 = local read "Small/HDPE 3"() -> (w1099:dbl)
                            n258 = Greater?(x=w1099, y=0.0) -> (0:w1100:bool)
                            n259 = case shown="True" w1100 {
                              frame False {
                                (unwired) "labview wouldnt let me copy the variables successfully\nso I had to write every single case structure by hand."
                              }
                              frame True {
                                n260 = local read "Small/HDPE 3"() -> (w1117:dbl)
                                n261 = xnode "Motors"() -> ("Motor"=w1101:T2)
                                n262 = Decrement(x=w1117) -> (x-1=w1116:dbl)
                                n263 = xnode "Move a Fixed Distance"("Speed 1"=i8 75, "Distance 1"=360, "Motors"=w1101) -> ("NXT/EV3"=w1104:T3)  [unwired: 1 in]
                                n264 = local write "Small/HDPE 3"(w1116) -> ()
                                n265 = xnode "Motors"() -> ("Motor"=w1105:T2)
                                n266 = xnode "Move a Fixed Distance"("Speed 1"=i8 -50, "Distance 1"=90, "Motors"=w1105, "NXT/EV3"=w1104) -> ("NXT/EV3"=w1115:T3)
                                n267 = xnode "Motors"() -> ("Motor"=w1111:T2)
                                n268 = xnode "Move a Fixed Distance"("Speed 1"=i8 -75, "Distance 1"=360, "Motors"=w1111, "NXT/EV3"=w1115) -> ("NXT/EV3"=w1114:T3)
                                n269 = xnode "Motors"() -> ("Motor"=w1108:T2)
                                n270 = xnode "Move a Fixed Distance"("Speed 1"=i8 50, "Distance 1"=90, "Motors"=w1108, "NXT/EV3"=w1114) -> ()  [unwired: 1 out]
                              }
                            }
                          }
                          frame True {
                            n271 = local read "Large/Steel 3"() -> (w1178:dbl)
                            n272 = Decrement(x=w1178) -> (x-1=w1177:dbl)
                            n273 = xnode "Motors"() -> ("Motor"=w1162:T2)
                            n274 = xnode "Move a Fixed Distance"("Speed 1"=i8 75, "Distance 1"=360, "Motors"=w1162) -> ("NXT/EV3"=w1165:T3)  [unwired: 1 in]
                            n275 = local write "Large/Steel 3"(w1177) -> ()
                            n276 = xnode "Motors"() -> ("Motor"=w1166:T2)
                            n277 = xnode "Move a Fixed Distance"("Speed 1"=i8 -50, "Distance 1"=90, "Motors"=w1166, "NXT/EV3"=w1165) -> ("NXT/EV3"=w1176:T3)
                            n278 = xnode "Motors"() -> ("Motor"=w1172:T2)
                            n279 = xnode "Move a Fixed Distance"("Speed 1"=i8 -75, "Distance 1"=360, "Motors"=w1172, "NXT/EV3"=w1176) -> ("NXT/EV3"=w1175:T3)
                            n280 = xnode "Motors"() -> ("Motor"=w1169:T2)
                            n281 = xnode "Move a Fixed Distance"("Speed 1"=i8 50, "Distance 1"=90, "Motors"=w1169, "NXT/EV3"=w1175) -> ()  [unwired: 1 out]
                          }
                        }
                      }
                    }
                  }
                }
              }
              frame True {
                n282 = local read "Material 2"() -> (w1223:string)
                n283 = case shown="\"Steel/HDPE\"" w1223 {
                  frame "White Glass", Default {
                    n284 = local read "Large/Steel 2"() -> (w1226:dbl)
                    n285 = Greater?(x=w1226, y=0.0) -> (0:w1224:bool)
                    n286 = case shown="False" w1224 {
                      frame False {
                        n287 = local read "Small/HDPE 2"() -> (w1229:dbl)
                        n288 = Greater?(x=w1229, y=0.0) -> (0:w1227:bool)
                        n289 = case shown="True" w1227 {
                          frame False {
                            (unwired) "howdy random TA"
                          }
                          frame True {
                            n290 = local read "Small/HDPE 2"() -> (w1246:dbl)
                            n291 = Decrement(x=w1246) -> (x-1=w1245:dbl)
                            n292 = local write "Small/HDPE 2"(w1245) -> ()
                            n293 = xnode "Motors"() -> ("Motor"=w1230:T2)
                            n294 = xnode "Move a Fixed Distance"("Speed 1"=i8 75, "Distance 1"=360, "Motors"=w1230) -> ("NXT/EV3"=w1233:T3)  [unwired: 1 in]
                            n295 = xnode "Motors"() -> ("Motor"=w1234:T2)
                            n296 = xnode "Move a Fixed Distance"("Speed 1"=i8 -50, "Distance 1"=90, "Motors"=w1234, "NXT/EV3"=w1233) -> ("NXT/EV3"=w1244:T3)
                            n297 = xnode "Motors"() -> ("Motor"=w1240:T2)
                            n298 = xnode "Move a Fixed Distance"("Speed 1"=i8 -75, "Distance 1"=360, "Motors"=w1240, "NXT/EV3"=w1244) -> ("NXT/EV3"=w1243:T3)
                            n299 = xnode "Motors"() -> ("Motor"=w1237:T2)
                            n300 = xnode "Move a Fixed Distance"("Speed 1"=i8 50, "Distance 1"=90, "Motors"=w1237, "NXT/EV3"=w1243) -> ()  [unwired: 1 out]
                          }
                        }
                      }
                      frame True {
                        n301 = local read "Large/Steel 2"() -> (w1307:dbl)
                        n302 = Decrement(x=w1307) -> (x-1=w1306:dbl)
                        n303 = local write "Large/Steel 2"(w1306) -> ()
                        n304 = xnode "Motors"() -> ("Motor"=w1291:T2)
                        n305 = xnode "Move a Fixed Distance"("Speed 1"=i8 75, "Distance 1"=360, "Motors"=w1291) -> ("NXT/EV3"=w1294:T3)  [unwired: 1 in]
                        n306 = xnode "Motors"() -> ("Motor"=w1295:T2)
                        n307 = xnode "Move a Fixed Distance"("Speed 1"=i8 -50, "Distance 1"=90, "Motors"=w1295, "NXT/EV3"=w1294) -> ("NXT/EV3"=w1305:T3)
                        n308 = xnode "Motors"() -> ("Motor"=w1301:T2)
                        n309 = xnode "Move a Fixed Distance"("Speed 1"=i8 -75, "Distance 1"=360, "Motors"=w1301, "NXT/EV3"=w1305) -> ("NXT/EV3"=w1304:T3)
                        n310 = xnode "Motors"() -> ("Motor"=w1298:T2)
                        n311 = xnode "Move a Fixed Distance"("Speed 1"=i8 50, "Distance 1"=90, "Motors"=w1298, "NXT/EV3"=w1304) -> ()  [unwired: 1 out]
                      }
                    }
                  }
                  frame "Blue Glass" {
                    n312 = local read "Large/Steel 2"() -> (w1354:dbl)
                    n313 = Greater?(x=w1354, y=0.0) -> (0:w1353:bool)
                    n314 = case shown="True" w1353 {
                      frame True {
                        n315 = local read "Large/Steel 2"() -> (w1371:dbl)
                        n316 = Decrement(x=w1371) -> (x-1=w1370:dbl)
                        n317 = local write "Large/Steel 2"(w1370) -> ()
                        n318 = xnode "Motors"() -> ("Motor"=w1355:T2)
                        n319 = xnode "Move a Fixed Distance"("Speed 1"=i8 75, "Distance 1"=360, "Motors"=w1355) -> ("NXT/EV3"=w1358:T3)  [unwired: 1 in]
                        n320 = xnode "Motors"() -> ("Motor"=w1359:T2)
                        n321 = xnode "Move a Fixed Distance"("Speed 1"=i8 -50, "Distance 1"=90, "Motors"=w1359, "NXT/EV3"=w1358) -> ("NXT/EV3"=w1369:T3)
                        n322 = xnode "Motors"() -> ("Motor"=w1365:T2)
                        n323 = xnode "Move a Fixed Distance"("Speed 1"=i8 -75, "Distance 1"=360, "Motors"=w1365, "NXT/EV3"=w1369) -> ("NXT/EV3"=w1368:T3)
                        n324 = xnode "Motors"() -> ("Motor"=w1362:T2)
                        n325 = xnode "Move a Fixed Distance"("Speed 1"=i8 50, "Distance 1"=90, "Motors"=w1362, "NXT/EV3"=w1368) -> ()  [unwired: 1 out]
                      }
                      frame False {
                        n326 = local read "Small/HDPE 2"() -> (w1418:dbl)
                        n327 = Greater?(x=w1418, y=0.0) -> (0:w1416:bool)
                        n328 = case shown="True" w1416 {
                          frame False {
                            (unwired) "This statement is false"
                          }
                          frame True {
                            n329 = local read "Small/HDPE 2"() -> (w1435:dbl)
                            n330 = Decrement(x=w1435) -> (x-1=w1434:dbl)
                            n331 = local write "Small/HDPE 2"(w1434) -> ()
                            n332 = xnode "Motors"() -> ("Motor"=w1419:T2)
                            n333 = xnode "Move a Fixed Distance"("Speed 1"=i8 75, "Distance 1"=360, "Motors"=w1419) -> ("NXT/EV3"=w1422:T3)  [unwired: 1 in]
                            n334 = xnode "Motors"() -> ("Motor"=w1423:T2)
                            n335 = xnode "Move a Fixed Distance"("Speed 1"=i8 -50, "Distance 1"=90, "Motors"=w1423, "NXT/EV3"=w1422) -> ("NXT/EV3"=w1433:T3)
                            n336 = xnode "Motors"() -> ("Motor"=w1429:T2)
                            n337 = xnode "Move a Fixed Distance"("Speed 1"=i8 -75, "Distance 1"=360, "Motors"=w1429, "NXT/EV3"=w1433) -> ("NXT/EV3"=w1432:T3)
                            n338 = xnode "Motors"() -> ("Motor"=w1426:T2)
                            n339 = xnode "Move a Fixed Distance"("Speed 1"=i8 50, "Distance 1"=90, "Motors"=w1426, "NXT/EV3"=w1432) -> ()  [unwired: 1 out]
                          }
                        }
                      }
                    }
                  }
                  frame "Red Glass" {
                    n340 = local read "Large/Steel 2"() -> (w1482:dbl)
                    n341 = Greater?(x=w1482, y=0.0) -> (0:w1480:bool)
                    n342 = case shown="False" w1480 {
                      frame False {
                        n343 = local read "Small/HDPE 2"() -> (w1485:dbl)
                        n344 = Greater?(x=w1485, y=0.0) -> (0:w1483:bool)
                        n345 = case shown="True" w1483 {
                          frame False {
                            (unwired) "I hate everything\n"
                          }
                          frame True {
                            n346 = local read "Small/HDPE 2"() -> (w1502:dbl)
                            n347 = xnode "Motors"() -> ("Motor"=w1486:T2)
                            n348 = xnode "Move a Fixed Distance"("Speed 1"=i8 75, "Distance 1"=360, "Motors"=w1486) -> ("NXT/EV3"=w1489:T3)  [unwired: 1 in]
                            n349 = Decrement(x=w1502) -> (x-1=w1501:dbl)
                            n350 = local write "Small/HDPE 2"(w1501) -> ()
                            n351 = xnode "Motors"() -> ("Motor"=w1490:T2)
                            n352 = xnode "Move a Fixed Distance"("Speed 1"=i8 -50, "Distance 1"=90, "Motors"=w1490, "NXT/EV3"=w1489) -> ("NXT/EV3"=w1500:T3)
                            n353 = xnode "Motors"() -> ("Motor"=w1496:T2)
                            n354 = xnode "Move a Fixed Distance"("Speed 1"=i8 -75, "Distance 1"=360, "Motors"=w1496, "NXT/EV3"=w1500) -> ("NXT/EV3"=w1499:T3)
                            n355 = xnode "Motors"() -> ("Motor"=w1493:T2)
                            n356 = xnode "Move a Fixed Distance"("Speed 1"=i8 50, "Distance 1"=90, "Motors"=w1493, "NXT/EV3"=w1499) -> ()  [unwired: 1 out]
                          }
                        }
                      }
                      frame True {
                        n357 = local read "Large/Steel 2"() -> (w1563:dbl)
                        n358 = Decrement(x=w1563) -> (x-1=w1562:dbl)
                        n359 = local write "Large/Steel 2"(w1562) -> ()
                        n360 = xnode "Motors"() -> ("Motor"=w1547:T2)
                        n361 = xnode "Move a Fixed Distance"("Speed 1"=i8 75, "Distance 1"=360, "Motors"=w1547) -> ("NXT/EV3"=w1550:T3)  [unwired: 1 in]
                        n362 = xnode "Motors"() -> ("Motor"=w1551:T2)
                        n363 = xnode "Move a Fixed Distance"("Speed 1"=i8 -50, "Distance 1"=90, "Motors"=w1551, "NXT/EV3"=w1550) -> ("NXT/EV3"=w1561:T3)
                        n364 = xnode "Motors"() -> ("Motor"=w1557:T2)
                        n365 = xnode "Move a Fixed Distance"("Speed 1"=i8 -75, "Distance 1"=360, "Motors"=w1557, "NXT/EV3"=w1561) -> ("NXT/EV3"=w1560:T3)
                        n366 = xnode "Motors"() -> ("Motor"=w1554:T2)
                        n367 = xnode "Move a Fixed Distance"("Speed 1"=i8 50, "Distance 1"=90, "Motors"=w1554, "NXT/EV3"=w1560) -> ()  [unwired: 1 out]
                      }
                    }
                  }
                  frame "Steel/HDPE" {
                    n368 = local read "Large/Steel 2"() -> (w1610:dbl)
                    n369 = Greater?(x=w1610, y=0.0) -> (0:w1608:bool)
                    n370 = case shown="True" w1608 {
                      frame False {
                        n371 = local read "Small/HDPE 2"() -> (w1613:dbl)
                        n372 = Greater?(x=w1613, y=0.0) -> (0:w1611:bool)
                        n373 = case shown="True" w1611 {
                          frame False {
                            (unwired) "I've lost all my marbles"
                          }
                          frame True {
                            n374 = local read "Small/HDPE 2"() -> (w1630:dbl)
                            n375 = xnode "Motors"() -> ("Motor"=w1614:T2)
                            n376 = xnode "Move a Fixed Distance"("Speed 1"=i8 75, "Distance 1"=360, "Motors"=w1614) -> ("NXT/EV3"=w1617:T3)  [unwired: 1 in]
                            n377 = Decrement(x=w1630) -> (x-1=w1629:dbl)
                            n378 = local write "Small/HDPE 2"(w1629) -> ()
                            n379 = xnode "Motors"() -> ("Motor"=w1618:T2)
                            n380 = xnode "Move a Fixed Distance"("Speed 1"=i8 -50, "Distance 1"=90, "Motors"=w1618, "NXT/EV3"=w1617) -> ("NXT/EV3"=w1628:T3)
                            n381 = xnode "Motors"() -> ("Motor"=w1624:T2)
                            n382 = xnode "Move a Fixed Distance"("Speed 1"=i8 -75, "Distance 1"=360, "Motors"=w1624, "NXT/EV3"=w1628) -> ("NXT/EV3"=w1627:T3)
                            n383 = xnode "Motors"() -> ("Motor"=w1621:T2)
                            n384 = xnode "Move a Fixed Distance"("Speed 1"=i8 50, "Distance 1"=90, "Motors"=w1621, "NXT/EV3"=w1627) -> ()  [unwired: 1 out]
                          }
                        }
                      }
                      frame True {
                        n385 = local read "Large/Steel 2"() -> (w1691:dbl)
                        n386 = Decrement(x=w1691) -> (x-1=w1690:dbl)
                        n387 = local write "Large/Steel 2"(w1690) -> ()
                        n388 = xnode "Motors"() -> ("Motor"=w1675:T2)
                        n389 = xnode "Move a Fixed Distance"("Speed 1"=i8 75, "Distance 1"=360, "Motors"=w1675) -> ("NXT/EV3"=w1678:T3)  [unwired: 1 in]
                        n390 = xnode "Motors"() -> ("Motor"=w1679:T2)
                        n391 = xnode "Move a Fixed Distance"("Speed 1"=i8 -50, "Distance 1"=90, "Motors"=w1679, "NXT/EV3"=w1678) -> ("NXT/EV3"=w1689:T3)
                        n392 = xnode "Motors"() -> ("Motor"=w1685:T2)
                        n393 = xnode "Move a Fixed Distance"("Speed 1"=i8 -75, "Distance 1"=360, "Motors"=w1685, "NXT/EV3"=w1689) -> ("NXT/EV3"=w1688:T3)
                        n394 = xnode "Motors"() -> ("Motor"=w1682:T2)
                        n395 = xnode "Move a Fixed Distance"("Speed 1"=i8 50, "Distance 1"=90, "Motors"=w1682, "NXT/EV3"=w1688) -> ()  [unwired: 1 out]
                      }
                    }
                  }
                }
              }
            }
          }
          frame True {
            n396 = local read "Material 1"() -> (w1736:string)
            n397 = case shown="\"Blue Glass\"" w1736 {
              frame "White Glass", Default {
                n398 = local read "Large/Steel 1"() -> (w1738:dbl)
                n399 = Greater?(x=w1738, y=0.0) -> (0:w1737:bool)
                n400 = case shown="False" w1737 {
                  frame False {
                    n401 = local read "Small/HDPE 1"() -> (w1741:dbl)
                    n402 = Greater?(x=w1741, y=0.0) -> (0:w1740:bool)
                    n403 = case shown="True" w1740 {
                      frame False {
                        (unwired) "go away"
                      }
                      frame True {
                        n404 = local read "Small/HDPE 1"() -> (w1759:dbl)
                        n405 = xnode "Motors"() -> ("Motor"=w1743:T2)
                        n406 = xnode "Move a Fixed Distance"("Speed 1"=i8 75, "Distance 1"=360, "Motors"=w1743) -> ("NXT/EV3"=w1746:T3)  [unwired: 1 in]
                        n407 = Decrement(x=w1759) -> (x-1=w1758:dbl)
                        n408 = local write "Small/HDPE 1"(w1758) -> ()
                        n409 = xnode "Motors"() -> ("Motor"=w1747:T2)
                        n410 = xnode "Move a Fixed Distance"("Speed 1"=i8 -50, "Distance 1"=90, "Motors"=w1747, "NXT/EV3"=w1746) -> ("NXT/EV3"=w1757:T3)
                        n411 = xnode "Motors"() -> ("Motor"=w1753:T2)
                        n412 = xnode "Move a Fixed Distance"("Speed 1"=i8 -75, "Distance 1"=360, "Motors"=w1753, "NXT/EV3"=w1757) -> ("NXT/EV3"=w1756:T3)
                        n413 = xnode "Motors"() -> ("Motor"=w1750:T2)
                        n414 = xnode "Move a Fixed Distance"("Speed 1"=i8 50, "Distance 1"=90, "Motors"=w1750, "NXT/EV3"=w1756) -> ()  [unwired: 1 out]
                      }
                    }
                  }
                  frame True {
                    n415 = local read "Large/Steel 1"() -> (w1820:dbl)
                    n416 = Decrement(x=w1820) -> (x-1=w1819:dbl)
                    n417 = local write "Large/Steel 1"(w1819) -> ()
                    n418 = xnode "Motors"() -> ("Motor"=w1804:T2)
                    n419 = xnode "Move a Fixed Distance"("Speed 1"=i8 75, "Distance 1"=360, "Motors"=w1804) -> ("NXT/EV3"=w1807:T3)  [unwired: 1 in]
                    n420 = xnode "Motors"() -> ("Motor"=w1808:T2)
                    n421 = xnode "Move a Fixed Distance"("Speed 1"=i8 -50, "Distance 1"=90, "Motors"=w1808, "NXT/EV3"=w1807) -> ("NXT/EV3"=w1818:T3)
                    n422 = xnode "Motors"() -> ("Motor"=w1814:T2)
                    n423 = xnode "Move a Fixed Distance"("Speed 1"=i8 -75, "Distance 1"=360, "Motors"=w1814, "NXT/EV3"=w1818) -> ("NXT/EV3"=w1817:T3)
                    n424 = xnode "Motors"() -> ("Motor"=w1811:T2)
                    n425 = xnode "Move a Fixed Distance"("Speed 1"=i8 50, "Distance 1"=90, "Motors"=w1811, "NXT/EV3"=w1817) -> ()  [unwired: 1 out]
                  }
                }
              }
              frame "Red Glass" {
                n426 = local read "Large/Steel 1"() -> (w1867:dbl)
                n427 = Greater?(x=w1867, y=0.0) -> (0:w1866:bool)
                n428 = case shown="False" w1866 {
                  frame False {
                    n429 = local read "Small/HDPE 1"() -> (w1870:dbl)
                    n430 = Greater?(x=w1870, y=0.0) -> (0:w1868:bool)
                    n431 = case shown="True" w1868 {
                      frame False {
                        (unwired) "donezo"
                      }
                      frame True {
                        n432 = xnode "Motors"() -> ("Motor"=w1871:T2)
                        n433 = local read "Small/HDPE 1"() -> (w1887:dbl)
                        n434 = xnode "Move a Fixed Distance"("Speed 1"=i8 75, "Distance 1"=360, "Motors"=w1871) -> ("NXT/EV3"=w1874:T3)  [unwired: 1 in]
                        n435 = Decrement(x=w1887) -> (x-1=w1886:dbl)
                        n436 = local write "Small/HDPE 1"(w1886) -> ()
                        n437 = xnode "Motors"() -> ("Motor"=w1875:T2)
                        n438 = xnode "Move a Fixed Distance"("Speed 1"=i8 -50, "Distance 1"=90, "Motors"=w1875, "NXT/EV3"=w1874) -> ("NXT/EV3"=w1885:T3)
                        n439 = xnode "Motors"() -> ("Motor"=w1881:T2)
                        n440 = xnode "Move a Fixed Distance"("Speed 1"=i8 -75, "Distance 1"=360, "Motors"=w1881, "NXT/EV3"=w1885) -> ("NXT/EV3"=w1884:T3)
                        n441 = xnode "Motors"() -> ("Motor"=w1878:T2)
                        n442 = xnode "Move a Fixed Distance"("Speed 1"=i8 50, "Distance 1"=90, "Motors"=w1878, "NXT/EV3"=w1884) -> ()  [unwired: 1 out]
                      }
                    }
                  }
                  frame True {
                    n443 = local read "Large/Steel 1"() -> (w1948:dbl)
                    n444 = xnode "Motors"() -> ("Motor"=w1932:T2)
                    n445 = Decrement(x=w1948) -> (x-1=w1947:dbl)
                    n446 = xnode "Move a Fixed Distance"("Speed 1"=i8 75, "Distance 1"=360, "Motors"=w1932) -> ("NXT/EV3"=w1935:T3)  [unwired: 1 in]
                    n447 = local write "Large/Steel 1"(w1947) -> ()
                    n448 = xnode "Motors"() -> ("Motor"=w1936:T2)
                    n449 = xnode "Move a Fixed Distance"("Speed 1"=i8 -50, "Distance 1"=90, "Motors"=w1936, "NXT/EV3"=w1935) -> ("NXT/EV3"=w1946:T3)
                    n450 = xnode "Motors"() -> ("Motor"=w1942:T2)
                    n451 = xnode "Move a Fixed Distance"("Speed 1"=i8 -75, "Distance 1"=360, "Motors"=w1942, "NXT/EV3"=w1946) -> ("NXT/EV3"=w1945:T3)
                    n452 = xnode "Motors"() -> ("Motor"=w1939:T2)
                    n453 = xnode "Move a Fixed Distance"("Speed 1"=i8 50, "Distance 1"=90, "Motors"=w1939, "NXT/EV3"=w1945) -> ()  [unwired: 1 out]
                  }
                }
              }
              frame "Blue Glass" {
                n454 = local read "Large/Steel 1"() -> (w1995:dbl)
                n455 = Greater?(x=w1995, y=0.0) -> (0:w1993:bool)
                n456 = case shown="True" w1993 {
                  frame False {
                    n457 = local read "Small/HDPE 1"() -> (w1997:dbl)
                    n458 = Greater?(x=w1997, y=0.0) -> (0:w1998:bool)
                    n459 = case shown="True" w1998 {
                      frame False {
                        (unwired) "Welcome to labview hell"
                      }
                      frame True {
                        n460 = local read "Small/HDPE 1"() -> (w2015:dbl)
                        n461 = xnode "Motors"() -> ("Motor"=w1999:T2)
                        n462 = xnode "Move a Fixed Distance"("Speed 1"=i8 75, "Distance 1"=360, "Motors"=w1999) -> ("NXT/EV3"=w2002:T3)  [unwired: 1 in]
                        n463 = Decrement(x=w2015) -> (x-1=w2014:dbl)
                        n464 = xnode "Motors"() -> ("Motor"=w2003:T2)
                        n465 = xnode "Move a Fixed Distance"("Speed 1"=i8 -50, "Distance 1"=90, "Motors"=w2003, "NXT/EV3"=w2002) -> ("NXT/EV3"=w2013:T3)
                        n466 = local write "Small/HDPE 1"(w2014) -> ()
                        n467 = xnode "Motors"() -> ("Motor"=w2009:T2)
                        n468 = xnode "Move a Fixed Distance"("Speed 1"=i8 -75, "Distance 1"=360, "Motors"=w2009, "NXT/EV3"=w2013) -> ("NXT/EV3"=w2012:T3)
                        n469 = xnode "Motors"() -> ("Motor"=w2006:T2)
                        n470 = xnode "Move a Fixed Distance"("Speed 1"=i8 50, "Distance 1"=90, "Motors"=w2006, "NXT/EV3"=w2012) -> ()  [unwired: 1 out]
                      }
                    }
                  }
                  frame True {
                    n471 = local read "Large/Steel 1"() -> (w2076:dbl)
                    n472 = xnode "Motors"() -> ("Motor"=w2060:T2)
                    n473 = xnode "Move a Fixed Distance"("Speed 1"=i8 75, "Distance 1"=360, "Motors"=w2060) -> ("NXT/EV3"=w2063:T3)  [unwired: 1 in]
                    n474 = Decrement(x=w2076) -> (x-1=w2075:dbl)
                    n475 = local write "Large/Steel 1"(w2075) -> ()
                    n476 = xnode "Motors"() -> ("Motor"=w2064:T2)
                    n477 = xnode "Move a Fixed Distance"("Speed 1"=i8 -50, "Distance 1"=90, "Motors"=w2064, "NXT/EV3"=w2063) -> ("NXT/EV3"=w2074:T3)
                    n478 = xnode "Motors"() -> ("Motor"=w2070:T2)
                    n479 = xnode "Move a Fixed Distance"("Speed 1"=i8 -75, "Distance 1"=360, "Motors"=w2070, "NXT/EV3"=w2074) -> ("NXT/EV3"=w2073:T3)
                    n480 = xnode "Motors"() -> ("Motor"=w2067:T2)
                    n481 = xnode "Move a Fixed Distance"("Speed 1"=i8 50, "Distance 1"=90, "Motors"=w2067, "NXT/EV3"=w2073) -> ()  [unwired: 1 out]
                  }
                }
              }
              frame "Steel/HDPE" {
                n482 = local read "Large/Steel 1"() -> (w2123:dbl)
                n483 = Greater?(x=w2123, y=0.0) -> (0:w2122:bool)
                n484 = case shown="False" w2122 {
                  frame False {
                    n485 = local read "Small/HDPE 1"() -> (w2126:dbl)
                    n486 = Greater?(x=w2126, y=0.0) -> (0:w2125:bool)
                    n487 = case shown="True" w2125 {
                      frame False {
                        (unwired) "why are you even here"
                      }
                      frame True {
                        n488 = local read "Small/HDPE 1"() -> (w2143:dbl)
                        n489 = xnode "Motors"() -> ("Motor"=w2127:T2)
                        n490 = Decrement(x=w2143) -> (x-1=w2142:dbl)
                        n491 = xnode "Move a Fixed Distance"("Speed 1"=i8 75, "Distance 1"=360, "Motors"=w2127) -> ("NXT/EV3"=w2130:T3)  [unwired: 1 in]
                        n492 = local write "Small/HDPE 1"(w2142) -> ()
                        n493 = xnode "Motors"() -> ("Motor"=w2131:T2)
                        n494 = xnode "Move a Fixed Distance"("Speed 1"=i8 -50, "Distance 1"=90, "Motors"=w2131, "NXT/EV3"=w2130) -> ("NXT/EV3"=w2141:T3)
                        n495 = xnode "Motors"() -> ("Motor"=w2137:T2)
                        n496 = xnode "Move a Fixed Distance"("Speed 1"=i8 -75, "Distance 1"=360, "Motors"=w2137, "NXT/EV3"=w2141) -> ("NXT/EV3"=w2140:T3)
                        n497 = xnode "Motors"() -> ("Motor"=w2134:T2)
                        n498 = xnode "Move a Fixed Distance"("Speed 1"=i8 50, "Distance 1"=90, "Motors"=w2134, "NXT/EV3"=w2140) -> ()  [unwired: 1 out]
                      }
                    }
                  }
                  frame True {
                    n499 = local read "Large/Steel 1"() -> (w2204:dbl)
                    n500 = Decrement(x=w2204) -> (x-1=w2203:dbl)
                    n501 = xnode "Motors"() -> ("Motor"=w2188:T2)
                    n502 = xnode "Move a Fixed Distance"("Speed 1"=i8 75, "Distance 1"=360, "Motors"=w2188) -> ("NXT/EV3"=w2191:T3)  [unwired: 1 in]
                    n503 = local write "Large/Steel 1"(w2203) -> ()
                    n504 = xnode "Motors"() -> ("Motor"=w2192:T2)
                    n505 = xnode "Move a Fixed Distance"("Speed 1"=i8 -50, "Distance 1"=90, "Motors"=w2192, "NXT/EV3"=w2191) -> ("NXT/EV3"=w2202:T3)
                    n506 = xnode "Motors"() -> ("Motor"=w2198:T2)
                    n507 = xnode "Move a Fixed Distance"("Speed 1"=i8 -75, "Distance 1"=360, "Motors"=w2198, "NXT/EV3"=w2202) -> ("NXT/EV3"=w2201:T3)
                    n508 = xnode "Motors"() -> ("Motor"=w2195:T2)
                    n509 = xnode "Move a Fixed Distance"("Speed 1"=i8 50, "Distance 1"=90, "Motors"=w2195, "NXT/EV3"=w2201) -> ()  [unwired: 1 out]
                  }
                }
              }
            }
          }
        }
      }
    }
  }
